vi "Search_Dust_Types.vi"() -> ()   [LabVIEW 2013]
uses:
  dust_list.ctl
panel:
  out "Descending":string
  out "Ascending":string
  out "dust_weight text":string
  out "bottle_weight text":string
  out "source_weight text":string
  out "dust_density text":string
  out "dust_name text":string
  out "id_dust_type text":string
  in  "Exit":bool
  out "error out":errorcluster
  in  "error in (no error)":errorcluster
  in  "dust_weight":bool
  in  "bottle_weight":bool
  in  "source_weight":bool
  in  "dust_density":bool
  in  "dust_name":bool
  in  "id_dust_type":bool
  out "Array":T1[](array[typedef])
  # "Size"
  # "Comments"
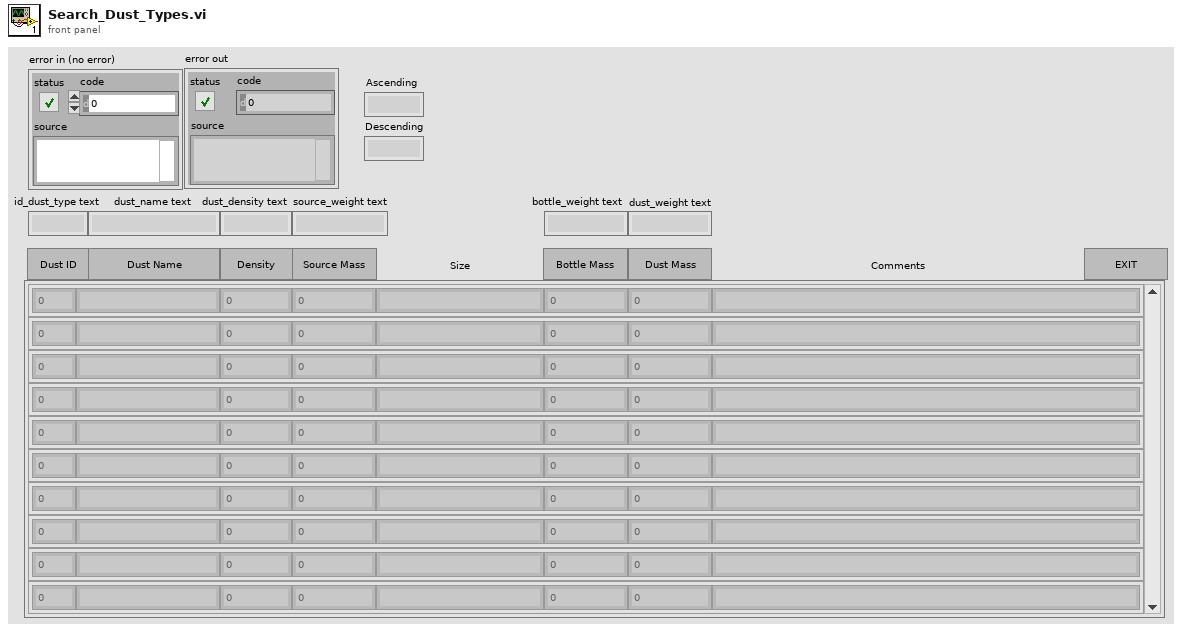
[diagram p1: front panel]
types:
  T1 = typedef "dust_list.ctl" = cluster{"id_dust_type":i32, "dust_name":string, "dust_density":dbl, "source_weight":dbl, "size":string, "bottle_weight":dbl, "dust_mass":dbl, "comments":string}
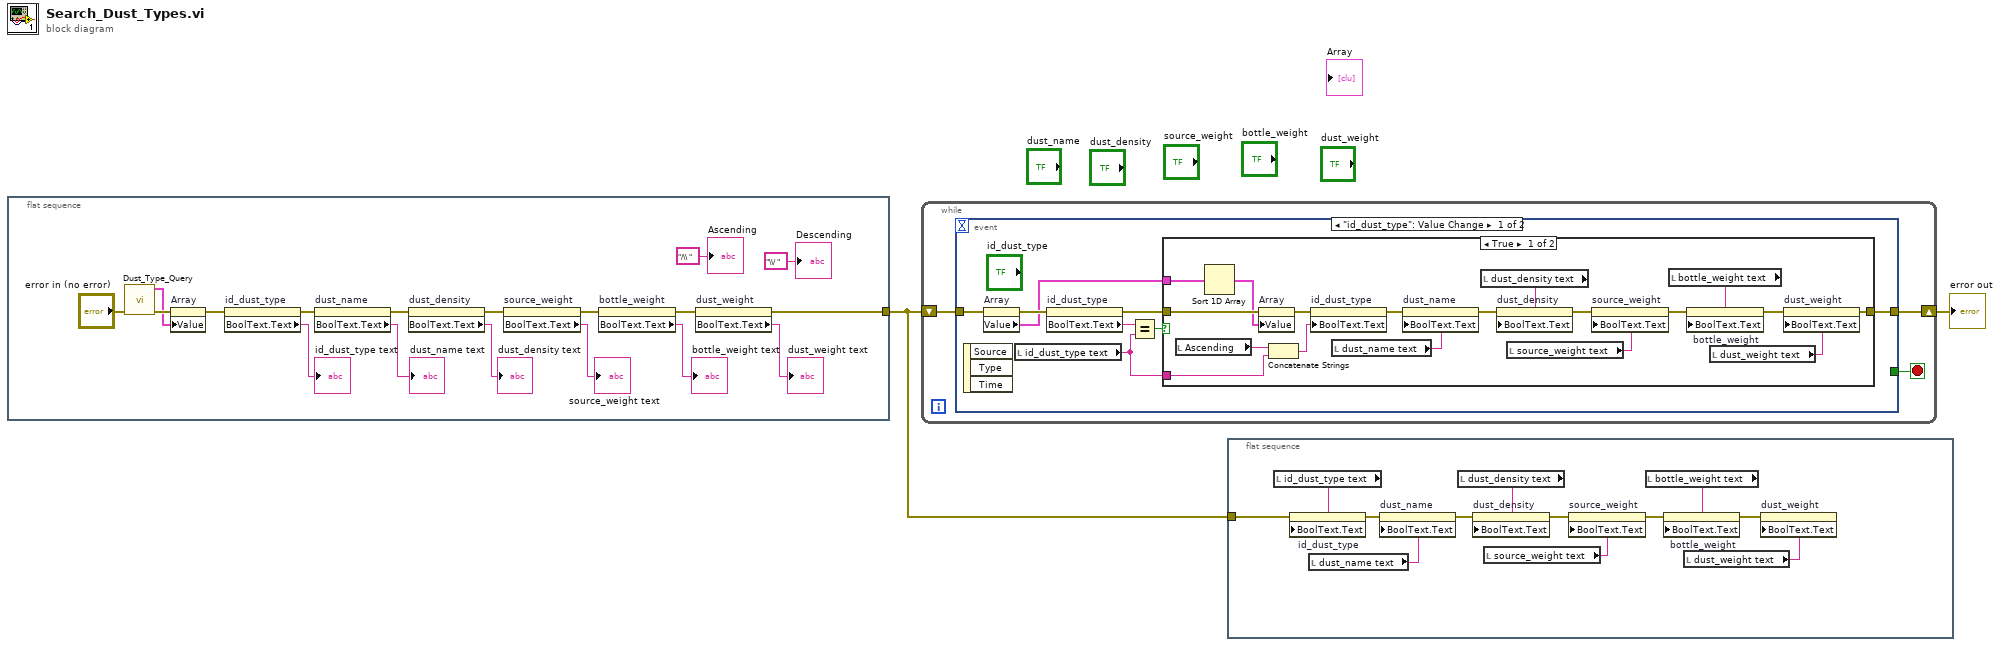
[diagram p0: block diagram]
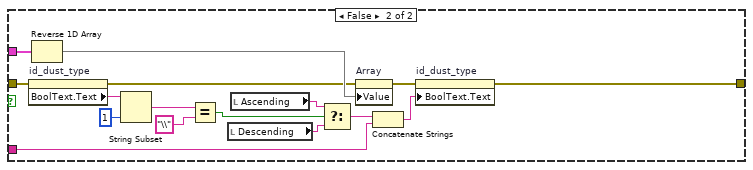
[diagram p2: hidden frame]
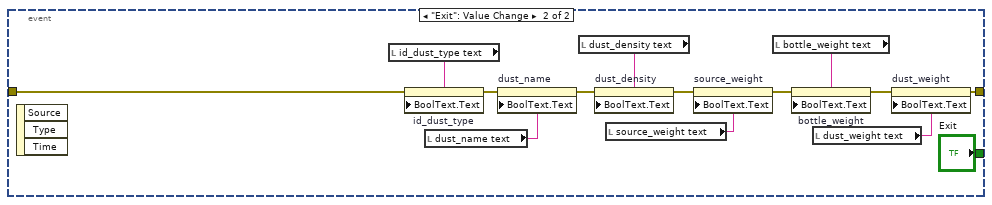
[diagram p3: hidden frame]
diagram:
  n1 = flat-sequence {
    tunnel: [w6] -> w1
    frame #0 {
      n2 = call "Dust_Type_Query.vi"("error in (no error)"="error in (no error)") -> ("error out"=w19:errorcluster, "Dust Type Array"=w18:T1[])  [unwired: 9 in]
      n3 = property on="Array" class="Arr (strict)"(error in=w19, "Value"=w18) -> (error out=w3:errorcluster)  [unwired: 1 in, 1 out]
      n4 = property on="id_dust_type" class="Bool"(error in=w3) -> (error out=w16:errorcluster, "BoolText.Text"=→"id_dust_type text":string)  [unwired: 1 in, 1 out]
      n5 = property on="dust_name" class="Bool"(error in=w16) -> (error out=w15:errorcluster, "BoolText.Text"=→"dust_name text":string)  [unwired: 1 in, 1 out]
      n6 = property on="dust_density" class="Bool"(error in=w15) -> (error out=w12:errorcluster, "BoolText.Text"=→"dust_density text":string)  [unwired: 1 in, 1 out]
      n7 = property on="source_weight" class="Bool"(error in=w12) -> (error out=w10:errorcluster, "BoolText.Text"=→"source_weight text":string)  [unwired: 1 in, 1 out]
      n8 = property on="bottle_weight" class="Bool"(error in=w10) -> (error out=w8:errorcluster, "BoolText.Text"=→"bottle_weight text":string)  [unwired: 1 in, 1 out]
      n9 = property on="dust_weight" class="Bool"(error in=w8) -> (error out=w6:errorcluster, "BoolText.Text"=→"dust_weight text":string)  [unwired: 1 in, 1 out]
      "Ascending" <- "/\\ " ("Ascending")
      "Descending" <- "\\/ " ("Descending")
    }
  }
  n10 = while {
    shift-right: [w22] -> w2
    shift-left: w1 -> [w23]
    stop <- w21 stop-if-true
    n11 = event shown="[0] \"id_dust_type\": Value Change" {
      selector: _ -> [_ _]
      dyn-events: _ -> [_ _]
      timeout: _ -> [_ _]
      tunnel: w23 -> [w31 w73]
      tunnel: [w30 w72] -> w22
      tunnel: [_ "Exit"] -> w21
      event "id_dust_type": Value Change {
        n12 = event-data() -> ()  [unwired: 1 in, 3 out]
        n13 = property on="Array" class="Arr (strict)"(error in=w31) -> (error out=w25:errorcluster, "Value"=w24:T1[])  [unwired: 1 in, 1 out]
        n14 = local read "id_dust_type text"() -> (w28:string)
        n15 = property on="id_dust_type" class="Bool"(error in=w25) -> (error out=w26:errorcluster, "BoolText.Text"=w29:string)  [unwired: 1 in, 1 out]
        n16 = Equal?(x=w29, y=w28) -> (x = y?=w27:bool)
        n17 = case shown="True" w27 {
          tunnel: [w36 w64] -> w30
          tunnel: w28 -> [w47 w63]
          tunnel: w26 -> [w35 w52]
          tunnel: w24 -> [w33 w62]
          frame True {
            n18 = local read "Ascending"() -> (w48:string)
            n19 = Sort 1D Array(array=w33) -> (sorted array=w32:T1[])
            n20 = property on="Array" class="Arr (strict)"(error in=w35, "Value"=w32) -> (error out=w34:errorcluster)  [unwired: 1 in, 1 out]
            n21 = Concatenate Strings(w48, w47) -> (w49:string)
            n22 = property on="id_dust_type" class="Bool"(error in=w34, "BoolText.Text"=w49) -> (error out=w37:errorcluster)  [unwired: 1 in, 1 out]
            n23 = local read "dust_name text"() -> (w41:string)
            n24 = property on="dust_name" class="Bool"(error in=w37, "BoolText.Text"=w41) -> (error out=w42:errorcluster)  [unwired: 1 in, 1 out]
            n25 = local read "dust_density text"() -> (w40:string)
            n26 = property on="dust_density" class="Bool"(error in=w42, "BoolText.Text"=w40) -> (error out=w43:errorcluster)  [unwired: 1 in, 1 out]
            n27 = local read "source_weight text"() -> (w39:string)
            n28 = property on="source_weight" class="Bool"(error in=w43, "BoolText.Text"=w39) -> (error out=w44:errorcluster)  [unwired: 1 in, 1 out]
            n29 = local read "bottle_weight text"() -> (w38:string)
            n30 = property on="bottle_weight" class="Bool"(error in=w44, "BoolText.Text"=w38) -> (error out=w45:errorcluster)  [unwired: 1 in, 1 out]
            n31 = local read "dust_weight text"() -> (w46:string)
            n32 = property on="dust_weight" class="Bool"(error in=w45, "BoolText.Text"=w46) -> (error out=w36:errorcluster)  [unwired: 1 in, 1 out]
          }
          frame False {
            n33 = property on="id_dust_type" class="Bool"(error in=w52) -> (error out=w51:errorcluster, "BoolText.Text"=w58:string)  [unwired: 1 in, 1 out]
            n34 = Reverse 1D Array(array=w62) -> (reversed array=w61:T1[])
            n35 = String Subset(string=w58, length (rest)=1 ("length (rest)")) -> (substring=w55:string)  [unwired: 1 in]
            n36 = Equal?(x=w55, y="\\") -> (x = y?=w53:bool)
            n37 = local read "Descending"() -> (w60:string)
            n38 = local read "Ascending"() -> (w56:string)
            n39 = Select(t=w56, s=w53, f=w60) -> (s? t:f=w59:string)
            n40 = property on="Array" class="Arr (strict)"(error in=w51, "Value"=w61) -> (error out=w50:errorcluster)  [unwired: 1 in, 1 out]
            n41 = Concatenate Strings(w59, w63) -> (w65:string)
            n42 = property on="id_dust_type" class="Bool"(error in=w50, "BoolText.Text"=w65) -> (error out=w64:errorcluster)  [unwired: 1 in, 1 out]
          }
        }
      }
      event "Exit": Value Change {
        n43 = event-data() -> ()  [unwired: 1 in, 3 out]
        n44 = local read "id_dust_type text"() -> (w71:string)
        n45 = property on="id_dust_type" class="Bool"(error in=w73, "BoolText.Text"=w71) -> (error out=w74:errorcluster)  [unwired: 1 in, 1 out]
        n46 = local read "dust_name text"() -> (w70:string)
        n47 = property on="dust_name" class="Bool"(error in=w74, "BoolText.Text"=w70) -> (error out=w75:errorcluster)  [unwired: 1 in, 1 out]
        n48 = local read "dust_density text"() -> (w69:string)
        n49 = property on="dust_density" class="Bool"(error in=w75, "BoolText.Text"=w69) -> (error out=w76:errorcluster)  [unwired: 1 in, 1 out]
        n50 = local read "source_weight text"() -> (w68:string)
        n51 = property on="source_weight" class="Bool"(error in=w76, "BoolText.Text"=w68) -> (error out=w77:errorcluster)  [unwired: 1 in, 1 out]
        n52 = local read "bottle_weight text"() -> (w67:string)
        n53 = property on="bottle_weight" class="Bool"(error in=w77, "BoolText.Text"=w67) -> (error out=w78:errorcluster)  [unwired: 1 in, 1 out]
        n54 = local read "dust_weight text"() -> (w66:string)
        n55 = property on="dust_weight" class="Bool"(error in=w78, "BoolText.Text"=w66) -> (error out=w72:errorcluster)  [unwired: 1 in, 1 out]
      }
    }
  }
  "error out" <- w2
  n56 = flat-sequence {
    tunnel: w1 -> [w80]
    frame #0 {
      n57 = local read "id_dust_type text"() -> (w87:string)
      n58 = property on="id_dust_type" class="Bool"(error in=w80, "BoolText.Text"=w87) -> (error out=w86:errorcluster)  [unwired: 1 in, 1 out]
      n59 = local read "dust_name text"() -> (w88:string)
      n60 = property on="dust_name" class="Bool"(error in=w86, "BoolText.Text"=w88) -> (error out=w85:errorcluster)  [unwired: 1 in, 1 out]
      n61 = local read "dust_density text"() -> (w89:string)
      n62 = property on="dust_density" class="Bool"(error in=w85, "BoolText.Text"=w89) -> (error out=w84:errorcluster)  [unwired: 1 in, 1 out]
      n63 = local read "source_weight text"() -> (w90:string)
      n64 = property on="source_weight" class="Bool"(error in=w84, "BoolText.Text"=w90) -> (error out=w83:errorcluster)  [unwired: 1 in, 1 out]
      n65 = local read "bottle_weight text"() -> (w91:string)
      n66 = property on="bottle_weight" class="Bool"(error in=w83, "BoolText.Text"=w91) -> (error out=w82:errorcluster)  [unwired: 1 in, 1 out]
      n67 = local read "dust_weight text"() -> (w81:string)
      n68 = property on="dust_weight" class="Bool"(error in=w82, "BoolText.Text"=w81) -> ()  [unwired: 1 in, 2 out]
    }
  }
